vi "Global.vi"() -> ()   [LabVIEW 2019]
panel:
  out "Path":path
  in  "Path Lenght":dbl=1.0
  in  "Lenght":i32=92
  in  "Start Index":i32=31
  in  "(220-240nm) Lenght":i32=36
  in  "(220-240nm) Index":i32=19
  in  "(240-260nm) Lenght":i32=37
  in  "(240-260nm) Index":i32=55
  out "I(TS)":dbl[](array[numeric])=[3792.125, 4026.0, 4170.875, 4454.375, 5068.875, 4951.875, 5250.75, 5623.375, 7564.5, 6369.875, 6787.75, 7202.125, 7539.625, 8041.125, 8308.875, 8723.0, 9100.375, 9664.625, 9859.625, 10374.375, 10712.0, 11207.5, 11627.125, 12592.5, 12599.5, 13215.5, 13790.75, 14442.375, 15098.25, 15884.125, 16883.625, 17471.125, 18205.0, 19212.5, 19992.5, 20907.125, 21761.875, 22635.875, 23614.25, 24291.75, 24861.125, 25720.25, 26124.0, 26296.5, 26530.0, 26689.375, 26670.0, 26690.25, 26553.0, 26425.125, 26129.375, 25922.875, 25612.125, 25247.25, 24874.375, 24521.25, 24146.25, 23904.25, 23506.75, 23284.875, 22950.0, 22638.125, 23171.625, 22257.625, 21792.125, 21529.25, 21252.75, 21084.625, 20896.125, 20872.875, 20794.75, 20949.625, 21090.375, 21539.125, 21748.0, 22067.5, 22450.75, 22889.25, 24823.25, 23391.625, 23390.625, 23431.125, 23221.5, 23087.5, 22902.5, 22995.25, 23142.375, 23382.625, 23695.875, 24269.625, 24355.75, 24562.375]
  out "I(KN)":dbl[](array[numeric])=[3738.625, 3976.75, 4069.5, 4233.875, 4871.75, 4714.5, 5012.375, 5379.75, 7255.75, 6048.125, 6446.25, 6844.5, 7209.625, 7756.875, 7962.25, 8423.25, 8827.25, 9437.75, 9637.625, 10217.5, 10609.5, 11152.125, 11594.875, 12660.875, 12733.875, 13412.875, 14012.75, 14724.375, 15394.875, 16225.75, 17321.75, 17957.625, 18807.5, 19783.375, 20627.625, 21629.5, 22474.875, 23415.75, 24410.25, 25156.875, 25682.625, 26583.125, 26983.125, 27186.75, 27397.0, 27544.375, 27519.375, 27515.375, 27334.625, 27168.375, 26883.75, 26611.25, 26257.625, 25866.25, 25511.75, 25111.875, 24731.25, 24491.625, 24080.625, 23800.375, 23475.375, 23189.875, 23672.375, 22750.5, 22265.625, 22039.5, 21698.25, 21547.25, 21364.875, 21289.5, 21241.875, 21437.125, 21545.875, 21983.625, 22233.5, 22597.375, 22992.25, 23420.875, 25387.625, 23959.625, 23961.25, 24026.0, 23794.625, 23703.375, 23568.125, 23624.375, 23777.0, 24088.375, 24416.375, 25033.375, 25127.375, 25347.625]
  out "I(ZN)":dbl[](array[numeric])=[3945.375, 4240.125, 4472.25, 4767.125, 5552.625, 5597.75, 6037.125, 6553.625, 8605.5, 7656.5, 8184.125, 8784.375, 9222.625, 9895.875, 10235.125, 10750.125, 11222.375, 11822.875, 12117.5, 12692.375, 13032.0, 13571.25, 14007.75, 14997.625, 15060.25, 15694.875, 16251.75, 16973.75, 17651.875, 18407.5, 19398.5, 19997.75, 20785.5, 21757.75, 22567.375, 23518.375, 24270.375, 25152.625, 26114.375, 26756.0, 27276.25, 28036.75, 28396.75, 28504.625, 28605.0, 28713.75, 28599.25, 28532.625, 28272.5, 28036.5, 27697.0, 27369.0, 27000.875, 26551.75, 26103.375, 25721.875, 25298.75, 25033.0, 24568.5, 24286.875, 23937.5, 23648.25, 24099.5, 23163.5, 22660.25, 22390.0, 22073.375, 21891.125, 21682.125, 21611.375, 21551.5, 21789.25, 21915.5, 22302.875, 22645.625, 22966.125, 23327.0, 23795.5, 25765.0, 24350.875, 24309.375, 24377.625, 24151.0, 24054.5, 23883.125, 23953.5, 24136.0, 24475.875, 24788.25, 25373.875, 25526.125, 25748.25]
  out "I(Blank)":dbl[](array[numeric])=[11528.875, 12086.875, 12417.875, 12768.75, 13472.875, 13329.375, 13485.875, 13646.625, 15258.875, 13815.125, 13888.25, 13986.0, 13962.625, 14176.75, 14089.875, 14216.5, 14311.375, 14651.625, 14599.875, 14939.25, 15120.25, 15440.0, 15700.875, 16594.5, 16538.875, 17080.75, 17621.25, 18222.5, 18850.5, 19606.5, 20602.375, 21225.75, 22006.875, 22994.25, 23773.375, 24692.625, 25497.0, 26407.75, 27343.875, 28025.25, 28535.5, 29313.75, 29649.625, 29755.5, 29937.125, 30004.125, 29871.5, 29807.75, 29541.5, 29300.5, 28893.875, 28570.625, 28191.25, 27721.5, 27245.75, 26825.0, 26401.375, 26085.875, 25653.125, 25324.5, 24950.375, 24633.0, 25069.125, 24148.125, 23600.375, 23352.375, 22998.5, 22823.5, 22571.75, 22489.875, 22454.875, 22640.75, 22748.125, 23197.125, 23516.25, 23876.375, 24264.5, 24763.375, 26737.375, 25303.0, 25317.375, 25341.625, 25096.625, 24986.0, 24825.875, 24858.125, 25048.125, 25356.375, 25740.75, 26341.375, 26497.375, 26730.375]
  out "I(Dark)":dbl[](array[numeric])=[2615.75, 2675.125, 2617.0, 2647.25, 3025.125, 2607.25, 2609.875, 2652.125, 4128.25, 2625.25, 2632.375, 2676.5, 2655.125, 2746.875, 2621.375, 2652.25, 2604.875, 2811.625, 2636.375, 2704.625, 2614.875, 2698.375, 2632.875, 3095.375, 2642.875, 2678.0, 2628.25, 2654.5, 2637.5, 2646.125, 2993.375, 2673.75, 2606.125, 2707.25, 2634.5, 2709.375, 2629.25, 2672.0, 2858.75, 2757.75, 2674.875, 2891.0, 2804.75, 2674.75, 2625.5, 2649.625, 2629.25, 2706.625, 2662.875, 2679.5, 2638.0, 2711.375, 2713.0, 2686.375, 2663.125, 2656.25, 2620.5, 2699.0, 2618.0, 2664.125, 2671.0, 2646.875, 3396.75, 2856.5, 2604.625, 2665.0, 2642.625, 2687.0, 2608.375, 2710.0, 2606.5, 2666.125, 2675.0, 2803.25, 2718.5, 2648.5, 2614.125, 2689.25, 4266.25, 2675.625, 2617.0, 2669.25, 2627.125, 2672.0, 2600.5, 2664.375, 2675.75, 2653.25, 2614.875, 2888.875, 2578.5, 2643.25]
  out "Lambda":dbl[](array[numeric])=[210.47, 211.013, 211.556, 212.099, 212.642, 213.185, 213.728, 214.271, 214.814, 215.357, 215.9, 216.443, 216.986, 217.529, 218.072, 218.615, 219.158, 219.701, 220.244, 220.787, 221.33, 221.873, 222.416, 222.959, 223.502, 224.045, 224.588, 225.131, 225.674, 226.217, 226.76, 227.303, 227.846, 228.389, 228.932, 229.475, 230.018, 230.561, 231.104, 231.647, 232.19, 232.733, 233.276, 233.819, 234.362, 234.905, 235.448, 235.991, 236.534, 237.077, 237.62, 238.163, 238.706, 239.249, 239.792, 240.335, 240.878, 241.421, 241.964, 242.507, 243.05, 243.593, 244.136, 244.679, 245.222, 245.765, 246.308, 246.851, 247.394, 247.937, 248.48, 249.023, 249.566, 250.109, 250.652, 251.195, 251.738, 252.281, 252.824, 253.367, 253.91, 254.453, 254.996, 255.539, 256.082, 256.625, 257.168, 257.711, 258.254, 258.797, 259.34, 259.883]
  in  "(210-260nm)Lenght":i32=92
  in  "(210-260nm) Index":i32
  in  "S(TS)":dbl=33.66
  in  "S(ZN)":dbl=36.052
  in  "S(KN)":dbl=33.85
  in  "S(Norm)":dbl=35.0
  in  "T(TS)":dbl=20.0
  in  "T(ZN)":dbl=19.3
  in  "T(KN)":dbl=21.0
  in  "[NO3-]":dbl=4.5e-05
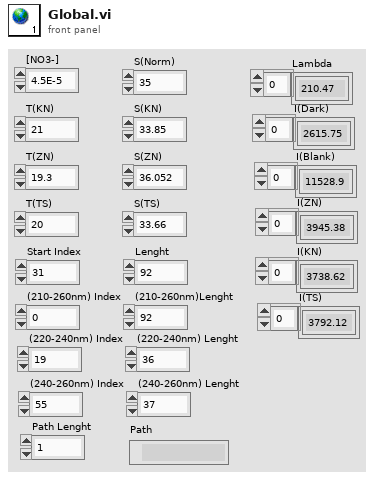
[diagram p1: front panel]
diagram:
